vi "ShellExecute.vi"(5 "show":i32(ring)=1 items=["SW_HIDE", "SW_SHOWNORMAL", "SW_SHOWMINIMIZED"], 6 "default directory":path, 7 "operation (open)":enum16{"open", "print"}(ring), 8 "error in (no error)":errorcluster, 9 "command line parameters":string, 10 "path to file":path, 11 "hWnd (NULL)":u32) -> (0 "error out":errorcluster)   [LabVIEW 2011]
doc: "This VI allows the user to either open or print a file as if it were selected from File Manager. Note that files whose extensions are not associated with an application will not be opened or printed.\n\nIf the VI is told to print a file, but the application that opens the file may not print a file, as dictated in the registration file, an error of -1027 is returned."
uses:
  SHELL32.DLL
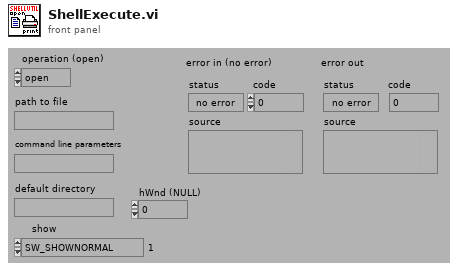
[diagram p1: front panel]
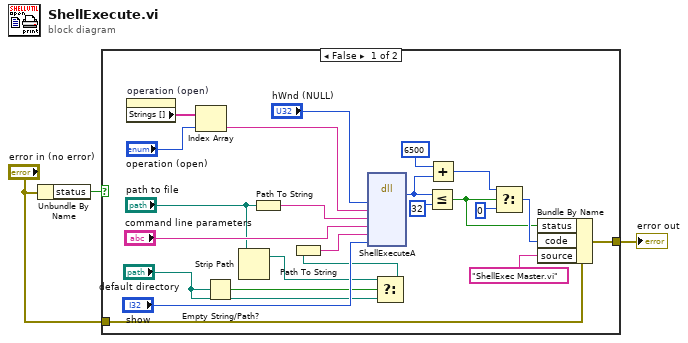
[diagram p0: block diagram]
diagram:
  n1 = Unbundle By Name("error in (no error)") -> ("status"=w3:bool)
  n2 = case shown="False" w3 {
    tunnel: "error in (no error)" -> [w12 w27]
    tunnel: [w11 w27] -> w1
    frame False {
      n3 = property on="operation (open)" class="Enum (strict)"() -> ("Strings []"=w20:string[])  [unwired: 2 in, 2 out]
      n4 = Index Array(array=w20, index="operation (open)") -> (element=w26:string)
      n5 = Empty String/Path?(string/path="default directory") -> (empty?=w8:bool)
      n6 = Strip Path(path="path to file") -> (stripped path=w4:path)  [unwired: 1 out]
      n7 = Path To String(path="path to file") -> (string=w25:string)
      n8 = Select(t=w4, s=w8, f="default directory") -> (s? t:f=w6:path)
      n9 = Path To String(path=w6) -> (string=w23:string)
      n10 = dll-call lib="SHELL32.DLL" fn="ShellExecuteA"("hWndParent"="hWnd (NULL)", "lpszOp"=w26, "lpszFile"=w25, "lpszParams"="command line parameters", "lpszDir"=w23, "fsShowCmd"="show") -> ("hInstance"=w16:u32)  [unwired: 8 in, 3 out]
      n11 = Less Or Equal?(x=w16, y=u16 32) -> (x <= y?=w13:bool)
      n12 = Add(x=6500, y=w16) -> (x+y=w10:u32)
      n13 = Select(t=w10, s=w13, f=0) -> (s? t:f=w14:u32)
      n14 = Bundle By Name(cluster=w12, "status"=w13, "code"=w14, "source"="ShellExec Master.vi") -> (w11:errorcluster)
    }
    frame True {
    }
  }
  "error out" <- w1
